vi "Handle Picture Mouse Down Event.vi"(7 "Button":u16, 8 "error in (no error)":errorcluster, 11 "dialog info in":T1={"steering frame ref"=refnum, "active wheel indexes"=[], "FP Refs"={"VI Refnum"=refnum, "Menu Ref"=refnum, "Sub Panel"=refnum, "picture"=refnum, "Steering Type"=refnum, "zoom in"=refnum, "zoom out"=refnum, "zoom extents"=refnum, "Wheels"=refnum, "Add Wheel"=refnum, "Remove Wheel"=refnum, "Copy Wheel"=refnum, "Angle Units"=refnum}, "subpanel info"={"subpanel VI refs"=[], "subpanel types"=[], "main to subpanel command events"=[]}, "picture dragging state"={"dragging"=FALSE, "wheel index"=-1, "dragging mode"=enum."translate", "wheel start position"={"x"=0.0, "y"=0.0, "theta"=0.0}, "relative mouse position"={"x"=0.0, "y"=0.0}, "relative mouse init angle (rad)"=0.0}, "picture size (pixels)"={"Width"=500, "Height"=500}, "picture grid"=bytes[0], "click zones group"={"click zones array"=[], "num click zones"=0}, "draw options"={"draw wheel states?"=FALSE, "highlight wheel index"=-1, "pixels per unit"=10.0, "draw forward velocity?"=FALSE, "velocity scale"=1.0}}) -> (0 "error out":errorcluster, 1 "discard?":bool, 3 "dialog info out":T1={"steering frame ref"=refnum, "active wheel indexes"=[], "FP Refs"={"VI Refnum"=refnum, "Menu Ref"=refnum, "Sub Panel"=refnum, "picture"=refnum, "Steering Type"=refnum, "zoom in"=refnum, "zoom out"=refnum, "zoom extents"=refnum, "Wheels"=refnum, "Add Wheel"=refnum, "Remove Wheel"=refnum, "Copy Wheel"=refnum, "Angle Units"=refnum}, "subpanel info"={"subpanel VI refs"=[], "subpanel types"=[], "main to subpanel command events"=[]}, "picture dragging state"={"dragging"=FALSE, "wheel index"=-1, "dragging mode"=enum."translate", "wheel start position"={"x"=0.0, "y"=0.0, "theta"=0.0}, "relative mouse position"={"x"=0.0, "y"=0.0}, "relative mouse init angle (rad)"=0.0}, "picture size (pixels)"={"Width"=500, "Height"=500}, "picture grid"=bytes[0], "click zones group"={"click zones array"=[], "num click zones"=0}, "draw options"={"draw wheel states?"=FALSE, "highlight wheel index"=-1, "pixels per unit"=10.0, "draw forward velocity?"=FALSE, "velocity scale"=1.0}})   [LabVIEW 2017, in "NI_Robotics_Configure Steering Frame.lvlib"]
uses:
  <vilib>/robotics/Dialog/Configure Steering Frame/NI_Robotics_Configure Steering Frame.lvlib
  <vilib>/robotics/Dialog/Configure Steering Frame/Dialog Info.ctl
  <vilib>/robotics/Steering/Steering Frame/NI_Robotics_Steering Frame.lvclass
  <vilib>/robotics/Dialog/Configure Steering Frame/FP Refs.ctl
  <vilib>/robotics/Dialog/Configure Steering Frame/Subpanel Info.ctl
  <vilib>/robotics/Dialog/Configure Steering Frame/Main to Subpanel Command Event.ctl
  <vilib>/robotics/Dialog/Configure Steering Frame/Main to Subpanel Command.ctl
  <vilib>/robotics/Dialog/Configure Steering Frame/Dragging State.ctl
  <vilib>/robotics/Dialog/Configure Steering Frame/Dragging Mode.ctl
  <vilib>/Utility/miscctls.llb/LVBoundsTypeDef.ctl
  <vilib>/robotics/Dialog/Configure Steering Frame/Click Zone.ctl
  <vilib>/robotics/Utilities/Visualization/Steering Visualization/Steering Picture/Draw Steering Frame Options.ctl
  <vilib>/Utility/cursorutil.llb/Set Cursor (Icon Pict).vi
  <vilib>/robotics/Dialog/Configure Steering Frame/Find Click Zone Wheel Index.vi
  <vilib>/robotics/Utilities/Visualization/Steering Visualization/Steering Picture/NI_Robotics_Steering Picture.lvlib
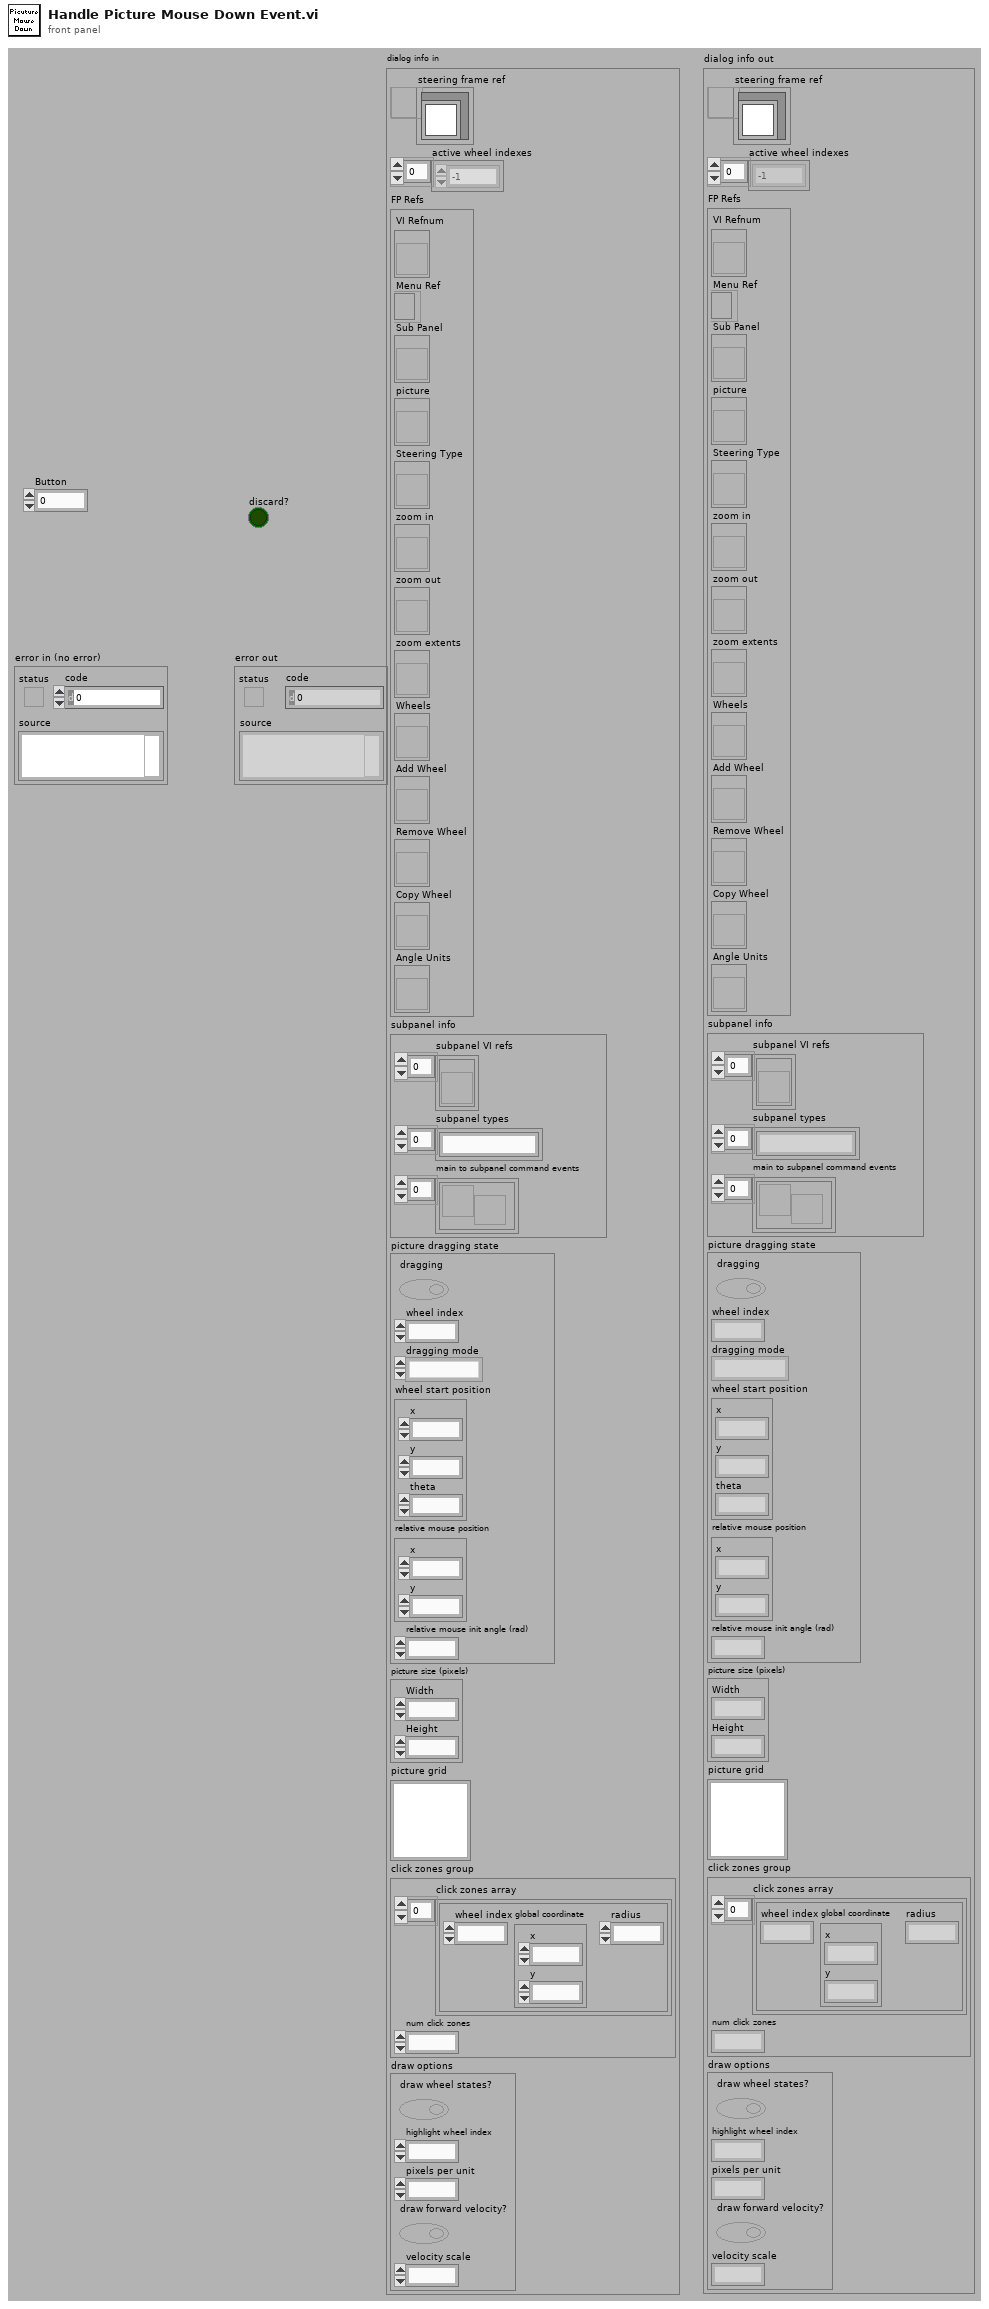
[diagram p1: front panel]
types:
  T1 = typedef "NI_Robotics_Configure Steering Frame.lvlib/Dialog Info.ctl" = cluster{"steering frame ref":refnum<data-value>, "active wheel indexes":i32[], "FP Refs":T2, "subpanel info":T3, "picture dragging state":T5, "picture size (pixels)":T7, "picture grid":picture, "click zones group":cluster{"click zones array":T8[], "num click zones":i32}, "draw options":T9}
  T2 = typedef "NI_Robotics_Configure Steering Frame.lvlib/FP Refs.ctl" = cluster{"VI Refnum":refnum<vi>, "Menu Ref":refnum<k9>, "Sub Panel":refnum<vi>, "picture":refnum<vi>, "Steering Type":refnum<vi>, "zoom in":refnum<vi>, "zoom out":refnum<vi>, "zoom extents":refnum<vi>, "Wheels":refnum<vi>, "Add Wheel":refnum<vi>, "Remove Wheel":refnum<vi>, "Copy Wheel":refnum<vi>, "Angle Units":refnum<vi>}
  T3 = typedef "NI_Robotics_Configure Steering Frame.lvlib/Subpanel Info.ctl" = cluster{"subpanel VI refs":refnum<vi>[], "subpanel types":string[], "main to subpanel command events":T4[]}
  T4 = typedef "NI_Robotics_Configure Steering Frame.lvlib/Main to Subpanel Command Event.ctl" = refnum<user-event>
  T5 = typedef "NI_Robotics_Configure Steering Frame.lvlib/Dragging State.ctl" = cluster{"dragging":bool, "wheel index":i32, "dragging mode":T6, "wheel start position":cluster{"x":dbl, "y":dbl, "theta":dbl}, "relative mouse position":cluster{"x":dbl, "y":dbl}, "relative mouse init angle (rad)":dbl}
  T6 = typedef "NI_Robotics_Configure Steering Frame.lvlib/Dragging Mode.ctl" = enum16{"translate", "rotate"}
  T7 = typedef "LVBoundsTypeDef.ctl" = cluster{"Width":u32, "Height":u32}
  T8 = typedef "NI_Robotics_Configure Steering Frame.lvlib/Click Zone.ctl" = cluster{"wheel index":i32, "global coordinate":cluster{"x":dbl, "y":dbl}, "radius":dbl}
  T9 = typedef "NI_Robotics_Steering Picture.lvlib/Draw Steering Frame Options.ctl" = cluster{"draw wheel states?":bool, "highlight wheel index":i32, "pixels per unit":dbl, "draw forward velocity?":bool, "velocity scale":dbl}
  T10 = typedef "LVMouseTypeDef.ctl" = cluster{"Mouse Position":cluster{"X":i32, "Y":i32}, "Mouse Modifiers":cluster{"Button Down":bool, "Shift Mod":bool, "Menu Mod":bool, "Option Mod":bool}}
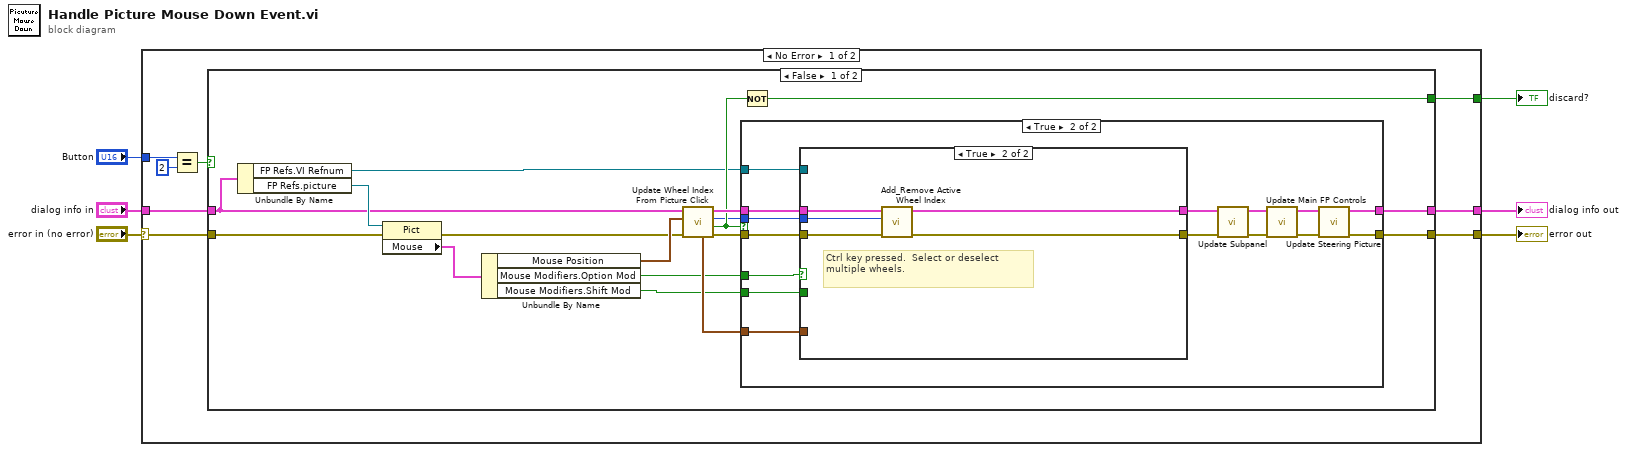
[diagram p0: block diagram]
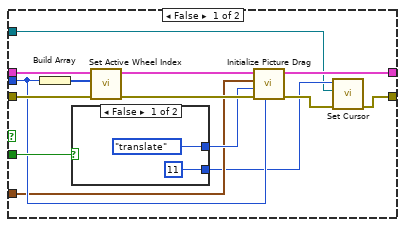
[diagram p3: hidden frame]
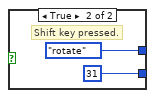
[diagram p4: hidden frame]
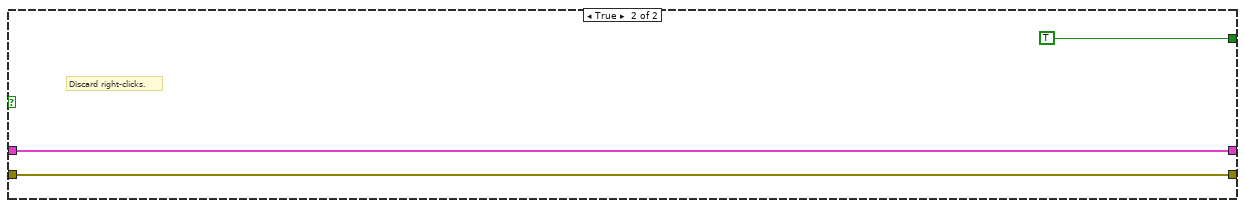
[diagram p5: hidden frame]
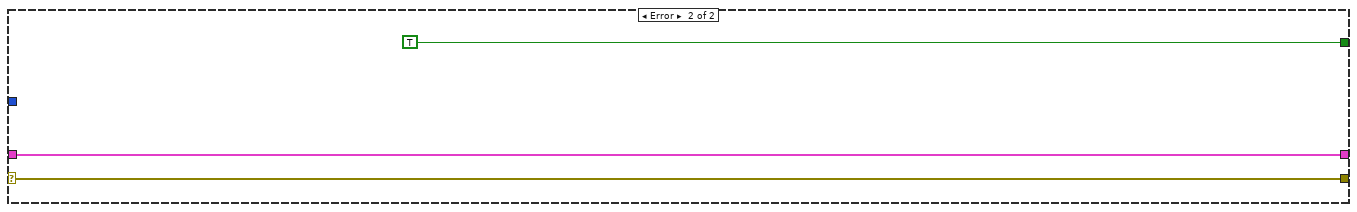
[diagram p6: hidden frame]
diagram:
  n1 = case shown="No Error" "error in (no error)" {
    selector: "error in (no error)" -> [w14 w76]
    tunnel: "dialog info in" -> [w13 w77]
    tunnel: [w12 w77] -> w4
    tunnel: [w11 w76] -> w3
    tunnel: [w10 TRUE] -> w2
    tunnel: "Button" -> [w9 _]
    frame No Error {
      n2 = Equal?(x=w9, y=u16 2) -> (x = y?=w7:bool)
      n3 = case shown="False" w7 {
        tunnel: w14 -> [w30 w72]
        tunnel: w13 -> [w24 w73]
        tunnel: [w23 w73] -> w12
        tunnel: [w22 w72] -> w11
        tunnel: [w20 TRUE] -> w10
        frame False {
          n4 = Unbundle By Name(w24) -> ("FP Refs.VI Refnum"=w18:refnum<vi>, "FP Refs.picture"=w31:refnum<vi>)
          n5 = property on="Property Node" class="Pict"(reference=w31, error in=w30) -> (error out=w26:errorcluster, "Mouse"=w25:T10)  [unwired: 1 out]
          n6 = Unbundle By Name(w25) -> ("Mouse Position"=w27:cluster{"X":i32, "Y":i32}, "Mouse Modifiers.Option Mod"=w15:bool, "Mouse Modifiers.Shift Mod"=w16:bool)
          n7 = call <vilib>:"Update Wheel Index From Picture Click.vi"("error in (no error)"=w26, "picture coordinate"=w27, "dialog info in"=w24) -> ("error out"=w28:errorcluster, "found?"=w21:bool, "selected wheel index"=w17:i32, "dialog info out"=w29:T1, "global mouse position"=w19:cluster{"x":dbl, "y":dbl})  [unwired: 4 in]
          n8 = case shown="True" w21 {
            tunnel: w29 -> [w33 w41]
            tunnel: [w33 w44] -> w23
            tunnel: w28 -> [w32 w39]
            tunnel: [w32 w43] -> w22
            tunnel: w19 -> [_ w35]
            tunnel: w18 -> [_ w34]
            tunnel: w17 -> [_ w37]
            tunnel: w16 -> [_ w42]
            tunnel: w15 -> [_ w36]
            frame False {
            }
            frame True {
              n9 = case shown="True" w36 {
                tunnel: w42 -> [w62 _]
                tunnel: w41 -> [w61 w71]
                tunnel: [w57 w70] -> w40
                tunnel: w39 -> [w60 w69]
                tunnel: [w51 w68] -> w38
                tunnel: w37 -> [w54 w67]
                tunnel: w35 -> [w53 _]
                tunnel: w34 -> [w49 _]
                frame False {
                  n10 = Build Array(w54) -> (w59:i32[])
                  n11 = case shown="False" w62 {
                    tunnel: [Dragging_Mode."translate" ("dragging mode") Dragging_Mode."rotate" ("dragging mode")] -> w55
                    tunnel: [u16 11 ("icon") u16 31 ("icon")] -> w50
                    frame False {
                    }
                    frame True {
                      # "Shift key pressed."
                    }
                  }
                  n12 = call <vilib>:"Set Active Wheel Index.vi"("error in (no error)"=w60, "active wheel indexes"=w59, "dialog info in"=w61) -> ("error out"=w56:errorcluster, "dialog info out"=w58:T1)  [unwired: 7 in]
                  n13 = call <vilib>:"Initialize Picture Drag.vi"("wheel index"=w54, "error in (no error)"=w56, "dragging mode"=w55, "global mouse position"=w53, "dialog info in"=w58) -> ("error out"=w52:errorcluster, "dialog info out"=w57:T1)  [unwired: 5 in]
                  n14 = call-poly <vilib>:"Set Cursor.vi"("error in (no error)"=w52, "VI reference (current VI)"=w49, "icon"=w50) -> ("error out"=w51:errorcluster)  [unwired: 7 in, 1 out]
                }
                frame True {
                  # "Ctrl key pressed.  Select or deselect multiple wheels."
                  n15 = call <vilib>:"Add_Remove Active Wheel Index.vi"("error in (no error)"=w69, "new active wheel index"=w67, "dialog info in"=w71) -> ("error out"=w68:errorcluster, "dialog info out"=w70:T1)  [unwired: 7 in]
                }
              }
              n16 = call <vilib>:"Update Subpanel.vi"("error in (no error)"=w38, "dialog info in"=w40) -> ("error out"=w45:errorcluster, "dialog info out"=w46:T1)  [unwired: 8 in]
              n17 = call <vilib>:"Update Main FP Controls.vi"("error in (no error)"=w45, "dialog info in"=w46) -> ("error out"=w47:errorcluster, "dialog info out"=w48:T1)  [unwired: 8 in]
              n18 = call <vilib>:"Update Steering Picture.vi"("error in (no error)"=w47, "dialog info in"=w48) -> ("error out"=w43:errorcluster, "dialog info out"=w44:T1)  [unwired: 8 in]
            }
          }
          n19 = Not(x=w21) -> (.not. x?=w20:bool)
        }
        frame True {
          # "Discard right-clicks."
        }
      }
    }
    frame Error {
    }
  }
  "error out" <- w3
  "dialog info out" <- w4
  "discard?" <- w2
